vi "write raw default value.vi"(8 "error in":errorcluster, 10 "raw default":variant, 11 "system tag in":refnum<class "data bus tag description.lvclass">) -> (0 "error out":errorcluster, 3 "system tag out":refnum<class "data bus tag description.lvclass">)   [LabVIEW 2013, in "data bus tag description.lvclass"]
doc: "Writes the default value field stored in the tag descriptor. This is a raw string, not an interpreted data type."
uses:
  data bus tag description.lvclass
  data bus tag description.lvclass/data bus tag description.ctl
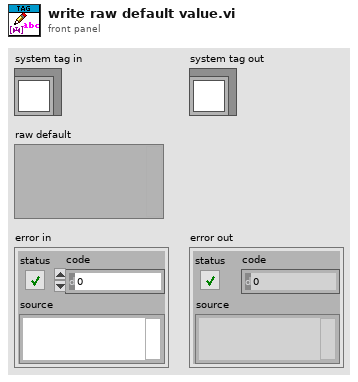
[diagram p1: front panel]
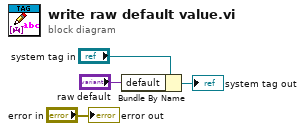
[diagram p0: block diagram]
diagram:
  n1 = Bundle By Name(cluster="system tag in", "default"="raw default") -> (→"system tag out":refnum<class "data bus tag description.lvclass">)
  "error out" <- "error in"
